vi "FG Waypoints reached.vi"(2 "FG Action (Read)":T1, 3 "Waypoints reached in":i8) -> (1 "Waypoints reached out":i8)   [LabVIEW 2009]
uses:
  Actions for FG's.ctl
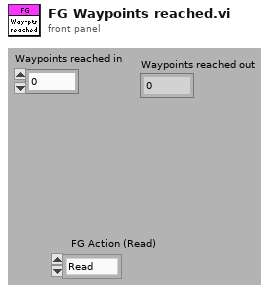
[diagram p1: front panel]
types:
  T1 = typedef "Actions for FG's.ctl" = enum16{"Read", "Write"}
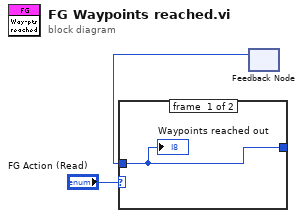
[diagram p0: block diagram]
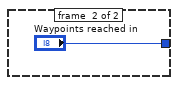
[diagram p2: hidden frame]
diagram:
  n1 = feedback #1() -> (w1:i8)  [unwired: 1 in]
  n2 = case shown="\"Write\"" "FG Action (Read)" {
    tunnel: [w4 "Waypoints reached in"] -> w2
    tunnel: w1 -> [w4 _]
    frame #0 {
      "Waypoints reached out" <- w4
    }
    frame #1 {
    }
  }
